vi "GOOP_StartObjectDebugger.vi"(1 "ClassToOpen":string, 5 "error in (no error)":errorcluster) -> (19 "error out":errorcluster)   [LabVIEW 2020]
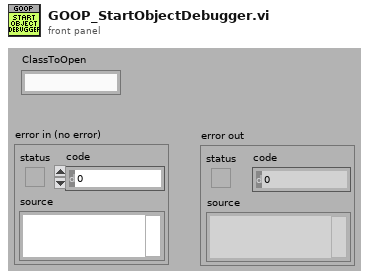
[diagram p1: front panel]
types:
  T1 = enum32{"Bad", "Idle", "Run top level", "Running"}
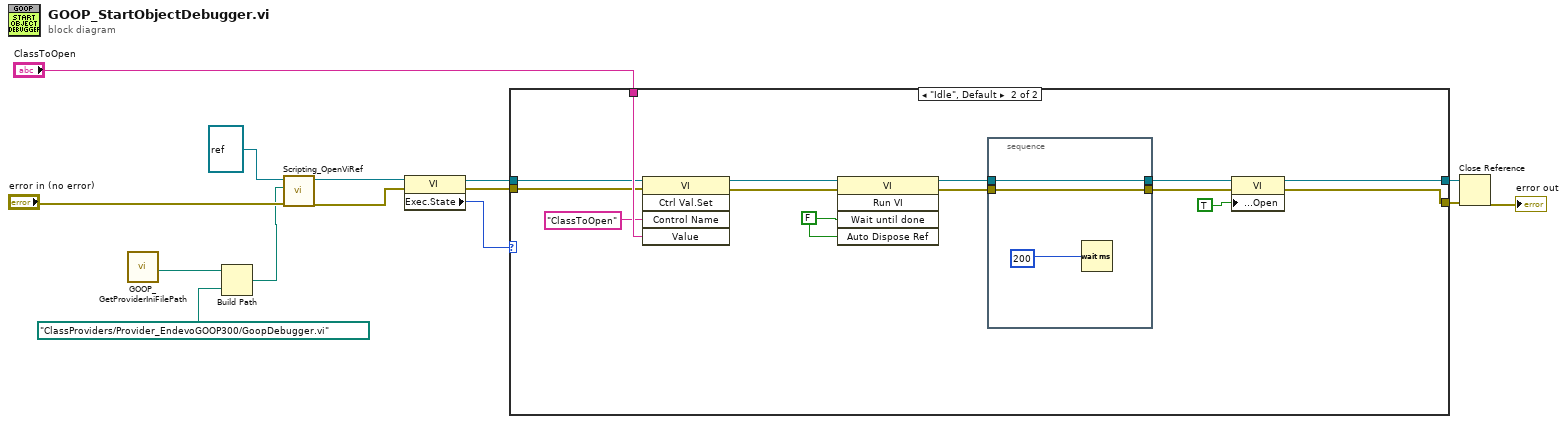
[diagram p0: block diagram]
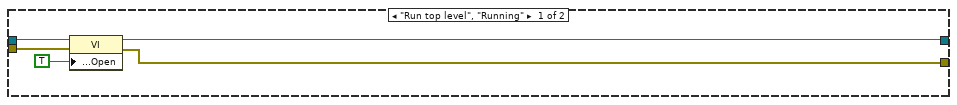
[diagram p2: hidden frame]
diagram:
  n1 = call <resource>:"GOOP_GetProviderIniFilePath.vi"() -> ("ProviderMainFolder"=w2:path)  [unwired: 10 in, 1 out]
  n2 = Build Path(base path=w2, name or relative path=path "ClassProviders/Provider_EndevoGOOP300/GoopDebugger.vi" ("base path")) -> (appended path=w10:path)
  n3 = call <resource>:"Scripting_OpenViRef.vi"("error in"="error in (no error)", "ViPath/ViName/Viref"=w10, "AppRef"=refnum<vi> refnum) -> ("error out"=w8:errorcluster, "vi reference"=w7:refnum<vi>)  [unwired: 6 in, 1 out]
  n4 = property class="VI"(reference=w7, error in=w8) -> (reference out=w5:refnum<vi>, error out=w6:errorcluster, "Exec.State"=w4:T1)
  n5 = case shown="\"Idle\", Default" w4 {
    tunnel: [w15 w22] -> w14
    tunnel: [w16 w23] -> w13
    tunnel: "ClassToOpen" -> [_ w33]
    tunnel: w6 -> [w18 w32]
    tunnel: w5 -> [w19 w31]
    frame "Run top level", "Running" {
      n6 = property class="VI"(reference=w19, error in=w18, "Front Panel.Open"=TRUE ("Front Panel Window:Open")) -> (reference out=w16:refnum<vi>, error out=w15:errorcluster)
    }
    frame "Idle", Default {
      w28 = FALSE ("Wait Until Done")
      n7 = invoke class="VI" method="Ctrl Val.Set"(reference=w31, error in=w32, "Control Name"="ClassToOpen" ("pattern"), "Value"=w33) -> (reference out=w26:refnum<vi>, error out=w25:errorcluster)  [unwired: 1 in, 3 out]
      n8 = invoke class="VI" method="Run VI"(reference=w26, error in=w25, "Wait until done"=w28, "Auto Dispose Ref"=w28) -> (reference out=w30:refnum<vi>, error out=w29:errorcluster)  [unwired: 1 in, 3 out]
      n9 = stacked-sequence {
        tunnel: w29 -> [w35]
        tunnel: w30 -> [w36]
        tunnel: [w36] -> w20
        tunnel: [w35] -> w21
        frame #0 {
          n10 = Wait (ms)(milliseconds to wait=200) -> ()  [unwired: 1 out]
        }
      }
      n11 = property class="VI"(reference=w20, error in=w21, "Front Panel.Open"=TRUE ("Front Panel Window:Open")) -> (reference out=w23:refnum<vi>, error out=w22:errorcluster)
    }
  }
  n12 = Close Reference(reference=w13, error in (no error)=w14) -> (error out=→"error out":errorcluster)
